vi "HTML Hierarhy Open.vi"(8 "error in (no error)":errorcluster) -> (0 "error out":errorcluster)   [LabVIEW 2014, in "lvprj2html.lvlib"]
uses:
  lvprj2html.lvlib
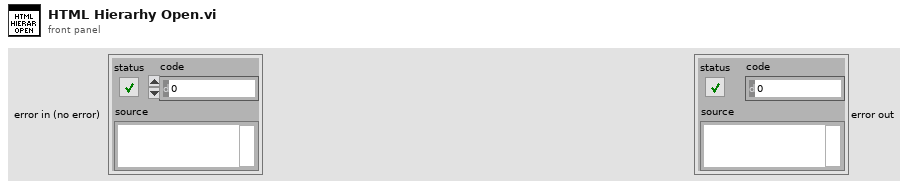
[diagram p1: front panel]
types:
  T1 = enum16{"open", "replace", "create", "open or create", "replace or create", "replace or create with confirmation"}
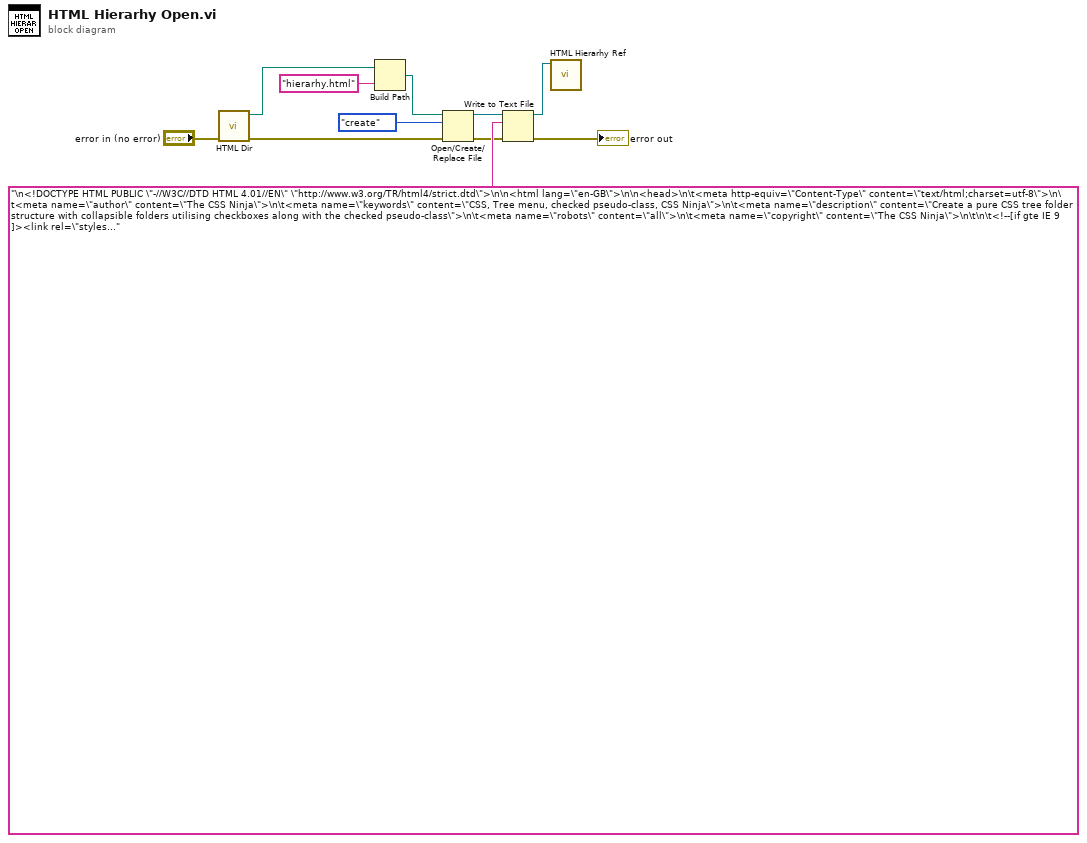
[diagram p0: block diagram]
diagram:
  n1 = call "HTML Dir.vi"("error in (no error)"="error in (no error)") -> ("error out"=w3:errorcluster, "path"=w5:path)  [unwired: 9 in]
  n2 = Build Path(base path=w5, name or relative path="hierarhy.html") -> (appended path=w7:path)
  n3 = Open/Create/Replace File(file path (use dialog)=w7, error in=w3, operation (0:open)=T1."create") -> (refnum out=w10:refnum<file>, error out=w2:errorcluster)  [unwired: 3 in, 1 out]
  n4 = Write to Text File(file (use dialog)=w10, text="\n<!DOCTYPE HTML PUBLIC \"-//W3C//DTD HTML 4.01//EN\" \"http://www.w3.org/TR/html4/strict.dtd\">\n\n<html lang=\"en-GB\">\n\n<head>\n\t<meta http-equiv=\"Content-Type\" content=\"text/html;charset=utf-8\">\n\t<meta name=\"author\" content=\"The CSS Ninja\">\n\t<meta name=\"keywords\" content=\"CSS, Tree menu, checked pseudo-class, CSS Ninja\">\n\t<meta name=\"description\" content=\"Create a pure CSS tree folder structure with collapsible folders utilising checkboxes along with the checked pseudo-class\">\n\t<meta name=\"robots\" content=\"all\">\n\t<meta name=\"copyright\" content=\"The CSS Ninja\">\n\t\n\t<!--[if gte IE 9 ]><link rel=\"stylesheet\" type=\"text/css\" href=\"../styles/styles.css\" media=\"screen\"><![endif]-->\n\t<!--[if !IE]>--><link rel=\"stylesheet\" type=\"text/css\" href=\"../styles/styles.css\" media=\"screen\"><!--<![endif]-->\n\t\n\t<title>Pure CSS collapsible tree menu | The CSS Ninja</title> \n \n</head>\n<body>\n\t\n\t<ol class=\"tree\">\n\t\n", error in=w2) -> (refnum out=w11:refnum<file>, error out=→"error out":errorcluster)  [unwired: 1 in, 1 out]
  n5 = call "HTML Hierarhy Ref.vi"("Byte Stream File in"=w11) -> ()  [unwired: 10 in, 1 out]
